vi "chooseKickTo.vi"(0 "KickToSkill in":refnum<class "KickToSkill.lvclass">, 1 "Game in":refnum<class "Game.lvclass">, 4 "target gap":dbl[](array[numeric]), 8 "Robot":refnum<class "Robot.lvclass">, 9 "KickForce 0?":bool, 10 "use criteria?":bool=TRUE, 11 "ForceInGame":bool, 12 "BadDribblerIDs":i32[](array[numeric]), 13 "pass?":bool, 15 "firstCall":bool, 16 "ChipKickInEnemyField":bool, 17 "Target":dbl[](array[numeric])) -> (20 "Game out":refnum<class "Game.lvclass">, 21 "Robot out":refnum<class "Robot.lvclass">)   [LabVIEW 2024, in "ShootTactic.lvclass"]
uses:
  ShootTactic.lvclass
  Game_class/Game.lvclass
  KickToSkill_class/KickToSkill.lvclass
  Robot_class/Robot.lvclass
  Robot_class/Robot.lvclass/Robot.ctl
  Robot_class/robotKickToStates.ctl
  Robot_class/Write robotKickState.vi
  Robot_class/Read id.vi
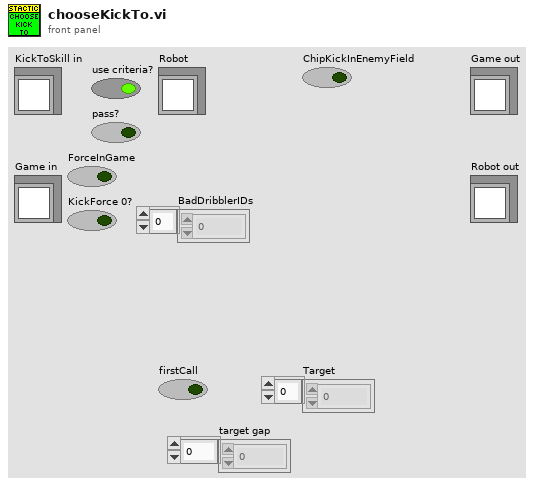
[diagram p1: front panel]
types:
  T1 = typedef "robotKickToStates.ctl" = enum16{"shootFromDirect", "avoidCollideBall", "goToBackBall", "none", "walk", "turn", "turnAntiClockWise", "turnClockwise", "oldKickToShoot", "oldKickToGoToBackBall", "shoot"}
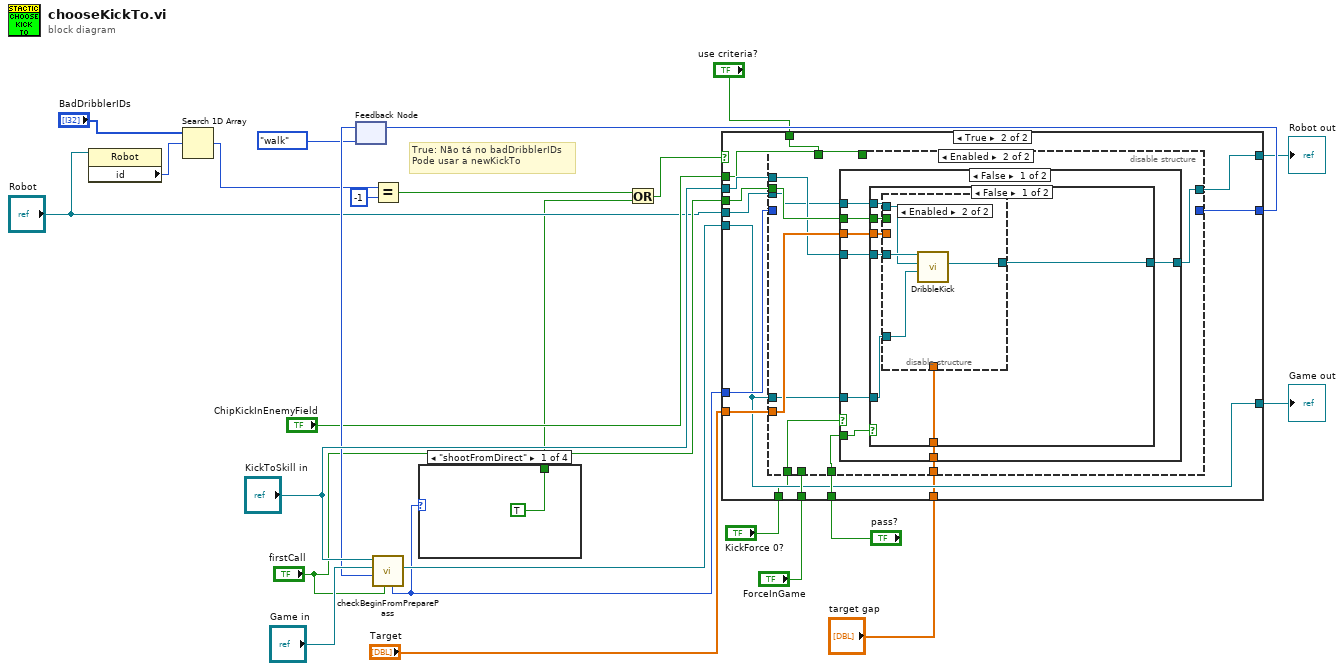
[diagram p0: block diagram]
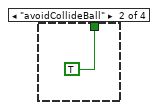
[diagram p2: hidden frame]
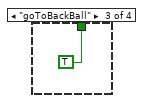
[diagram p3: hidden frame]
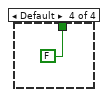
[diagram p4: hidden frame]
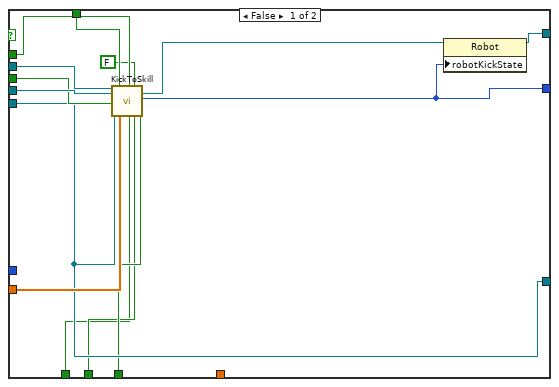
[diagram p5: hidden frame]
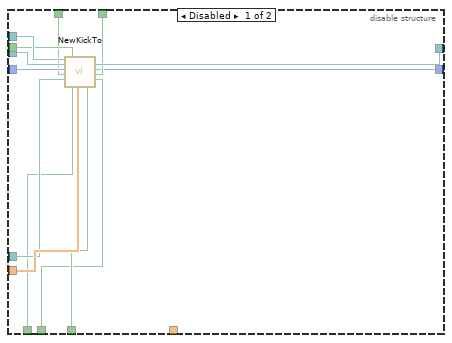
[diagram p6: hidden frame]
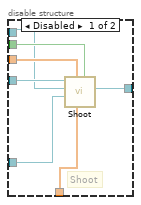
[diagram p7: hidden frame]
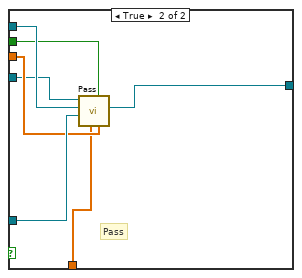
[diagram p8: hidden frame]
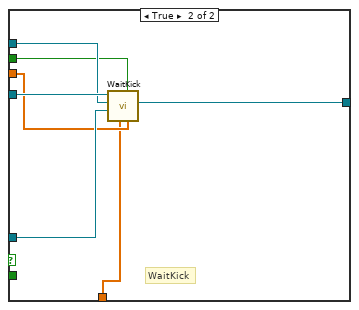
[diagram p9: hidden frame]
diagram:
  # "True: Não tá no badDribblerIDs\nPode usar a newKickTo"
  n1 = property class="Robot"(reference="Robot") -> ("id"=w8:i32)  [unwired: 1 in, 2 out]
  n2 = Search 1D Array(1D array="BadDribblerIDs", element=w8) -> (index of element=w7:i32)  [unwired: 1 in]
  n3 = feedback #1(robotKickToStates."walk" ("robotKickState")) -> (w21:T1)
  n4 = Equal?(x=w7, y=-1) -> (x = y?=w5:bool)
  n5 = call "checkBeginFromPreparePass.vi"("firstCall?"="firstCall", "robotKickState in"=w21, "Game in"="Game in", "KickToSkill in"="KickToSkill in") -> ("Game out"=w24:refnum<class "Game.lvclass">, "state out"=w4:T1)  [unwired: 3 in, 3 out]
  n6 = case shown="\"shootFromDirect\"" w4 {
    tunnel: [TRUE TRUE TRUE FALSE] -> w3
    frame "shootFromDirect" {
    }
    frame "avoidCollideBall" {
    }
    frame "goToBackBall" {
    }
    frame Default {
    }
  }
  n7 = Or(x=w5, y=w3) -> (x .or. y?=w6:bool)
  n8 = case shown="True" w6 {
    tunnel: "KickToSkill in" -> [w39 w57]
    tunnel: [w32 w56] -> w15
    tunnel: "Robot" -> [w43 w55]
    tunnel: "Target" -> [w41 w54]
    tunnel: w24 -> [w40 w46]
    tunnel: "firstCall" -> [w42 w53]
    tunnel: [w40 w46] -> w17
    tunnel: "ChipKickInEnemyField" -> [w38 w52]
    tunnel: w4 -> [_ w51]
    tunnel: [w31 w50] -> w25
    tunnel: "pass?" -> [w37 w48]
    tunnel: "ForceInGame" -> [w36 w47]
    tunnel: "KickForce 0?" -> [w35 w45]
    tunnel: "use criteria?" -> [w34 w49]
    tunnel: "target gap" -> [_ w44]
    frame False {
      n9 = call "KickToSkill.vi"("KickToSkill in"=w39, "Robot"=w43, "firstCall?"=w42, "Game"=w40, "use criteria?"=w34, "Target"=w41, "chipKick ?"=w38, "KickForce 0?"=w35, "WeakKick"=FALSE, "ForceInGame"=w36, "pass?"=w37) -> ("Robot out"=w33:refnum<class "Robot.lvclass">, "robotKickState out"=w31:T1)  [unwired: 5 in, 2 out]
      n10 = property class="Robot"(reference=w33, "robotKickState"=w31) -> (reference out=w32:refnum<class "Robot.lvclass">)  [unwired: 1 in, 1 out]
    }
    frame True {
      n11 = disable-structure shown="Enabled" {
        disable-tunnel: w57 -> [w70 w75]
        disable-tunnel: [w69 w72] -> w56
        disable-tunnel: w55 -> [w68 w74]
        disable-tunnel: w54 -> [w67 w77]
        disable-tunnel: w53 -> [w66 w76]
        disable-tunnel: w52 -> [w65 _]
        disable-tunnel: w51 -> [w64 _]
        disable-tunnel: [w63 _] -> w50
        disable-tunnel: w49 -> [w62 _]
        disable-tunnel: w48 -> [w61 w78]
        disable-tunnel: w47 -> [w60 _]
        disable-tunnel: w46 -> [w59 w73]
        disable-tunnel: w45 -> [w58 w79]
        disable-tunnel: w44 -> [_ w71]
        frame Disabled {
          n12 = call "NewKickTo.vi"("KickToSkill in"=w70, "Robot"=w68, "State in"=w64, "use criteria?"=w62, "Game"=w59, "firstCall?"=w66, "kickforce0?"=w58, "Target"=w67, "pass?"=w61, "chipKick ?"=w65, "ForceInGame"=w60) -> ("Robot out"=w69:refnum<class "Robot.lvclass">, "State out"=w63:T1)  [unwired: 5 in, 2 out]
        }
        frame Enabled {
          n13 = case shown="False" w79 {
            tunnel: w78 -> [w87 _]
            tunnel: w77 -> [w86 w114]
            tunnel: w76 -> [w85 w115]
            tunnel: w75 -> [w84 w119]
            tunnel: w74 -> [w83 w117]
            tunnel: w73 -> [w82 w116]
            tunnel: [w81 w118] -> w72
            tunnel: w71 -> [w80 w113]
            frame False {
              n14 = case shown="False" w87 {
                tunnel: w86 -> [w94 w108]
                tunnel: w85 -> [w93 w110]
                tunnel: w84 -> [w92 w107]
                tunnel: w83 -> [w91 w112]
                tunnel: w82 -> [w90 w109]
                tunnel: [w89 w111] -> w81
                tunnel: w80 -> [w88 w106]
                frame False {
                  n15 = disable-structure shown="Enabled" {
                    disable-tunnel: w94 -> [w101 _]
                    disable-tunnel: w93 -> [w100 _]
                    disable-tunnel: w92 -> [w99 w105]
                    disable-tunnel: w91 -> [w98 w104]
                    disable-tunnel: w90 -> [w97 w103]
                    disable-tunnel: [w96 w102] -> w89
                    disable-tunnel: w88 -> [w95 _]
                    frame Disabled {
                      # "Shoot"
                      n16 = call "Shoot.vi"("FirstCall?"=w100, "target gap"=w95, "KickTarget"=w101, "Game"=w97, "Robot"=w98, "KickToSkill in"=w99) -> ("Robot out"=w96:refnum<class "Robot.lvclass">)  [unwired: 3 in, 2 out]
                    }
                    frame Enabled {
                      n17 = call "DribbleKick.vi"("Game"=w103, "Robot"=w104, "KickToSkill in"=w105) -> ("Robot out"=w102:refnum<class "Robot.lvclass">)  [unwired: 6 in, 2 out]
                    }
                  }
                }
                frame True {
                  # "Pass"
                  n18 = call "Pass.vi"("KickTarget"=w108, "firstCall?"=w110, "target gap"=w106, "Game"=w109, "Robot"=w112, "KickToSkill in"=w107) -> ("Robot out"=w111:refnum<class "Robot.lvclass">)  [unwired: 3 in, 2 out]
                }
              }
            }
            frame True {
              # "WaitKick"
              n19 = call "WaitKick.vi"("KickTarget"=w114, "firstCall?"=w115, "target gap"=w113, "Game"=w116, "Robot"=w117, "KickToSkill in"=w119) -> ("Robot out"=w118:refnum<class "Robot.lvclass">)  [unwired: 3 in, 2 out]
            }
          }
        }
      }
    }
  }
  "Game out" <- w17
  "Robot out" <- w15
  n20 = feedback-in #1(w25) -> ()
